vi "WaveGenerator.vi"(0 "Data array":dbl[][](array[numeric]), 1 "dt":dbl, 3 "TestLoops":i32, 5 "VMIC command":dbl[](array[numeric]), 9 "WaveDefineArray":T1[](array[typedef]) {"Enable" items=["不使能", "使能"]; "Wave" items=["0指令", "正弦波", "方波", "三角波", "常值", "波形数据", "白噪声", "正弦扫频", "梯度加载", "VMIC"]; "ChannelType" items=["标准波形跟踪"=1, "扫频测试"=2, "消除多余力"=3, "梯度加载"=4, "载荷谱跟踪"=5, "模拟输入跟踪"=9]; "ChannelStatus" items=["通道关", "位置通道", "加载通道"]}, 11 "Angle":dbl[](array[numeric]), 12 "AxisForce":dbl[](array[numeric]), 14 "LastVMICcommand":dbl[](array[numeric])) -> (4 "wave out 2":dbl[](array[numeric]), 6 "Command":dbl[](array[numeric]), 10 "Boolean":bool, 13 "VMICafterFilter":dbl[](array[numeric]), 15 "type out":dbl[](array[numeric]))   [LabVIEW 2014]
uses:
  ChannelCommand.ctl
  Control 1.ctl
  WaveType.ctl
  MoterEnable.ctl
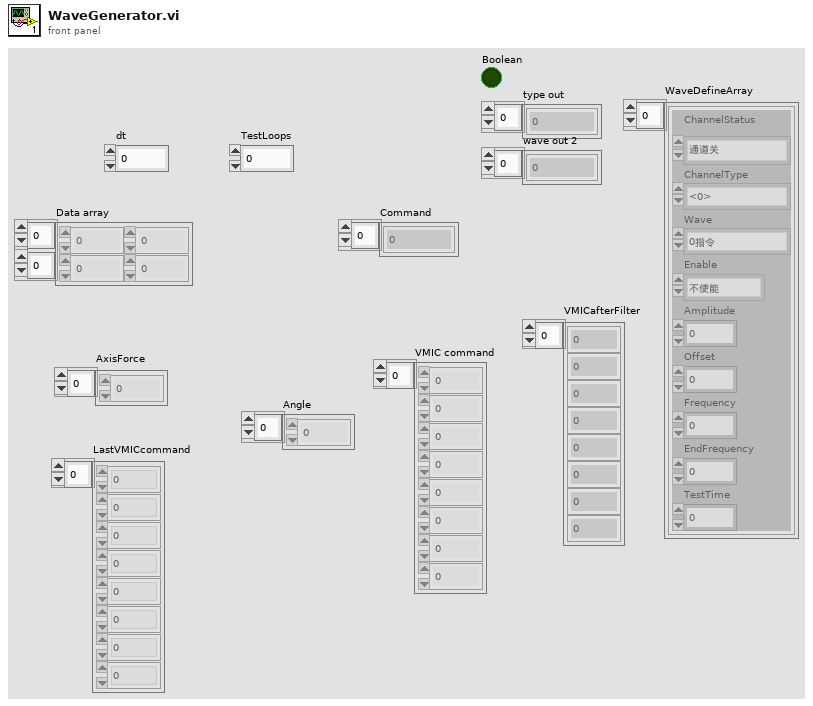
[diagram p1: front panel]
types:
  T1 = typedef "ChannelCommand.ctl" = cluster{"ChannelStatus":T2, "ChannelType":i32, "Wave":T3, "Enable":T4, "Amplitude":dbl, "Offset":dbl, "Frequency":dbl, "EndFrequency":dbl, "TestTime":dbl}
  T2 = typedef "Control 1.ctl" = i32
  T3 = typedef "WaveType.ctl" = i32
  T4 = typedef "MoterEnable.ctl" = u16
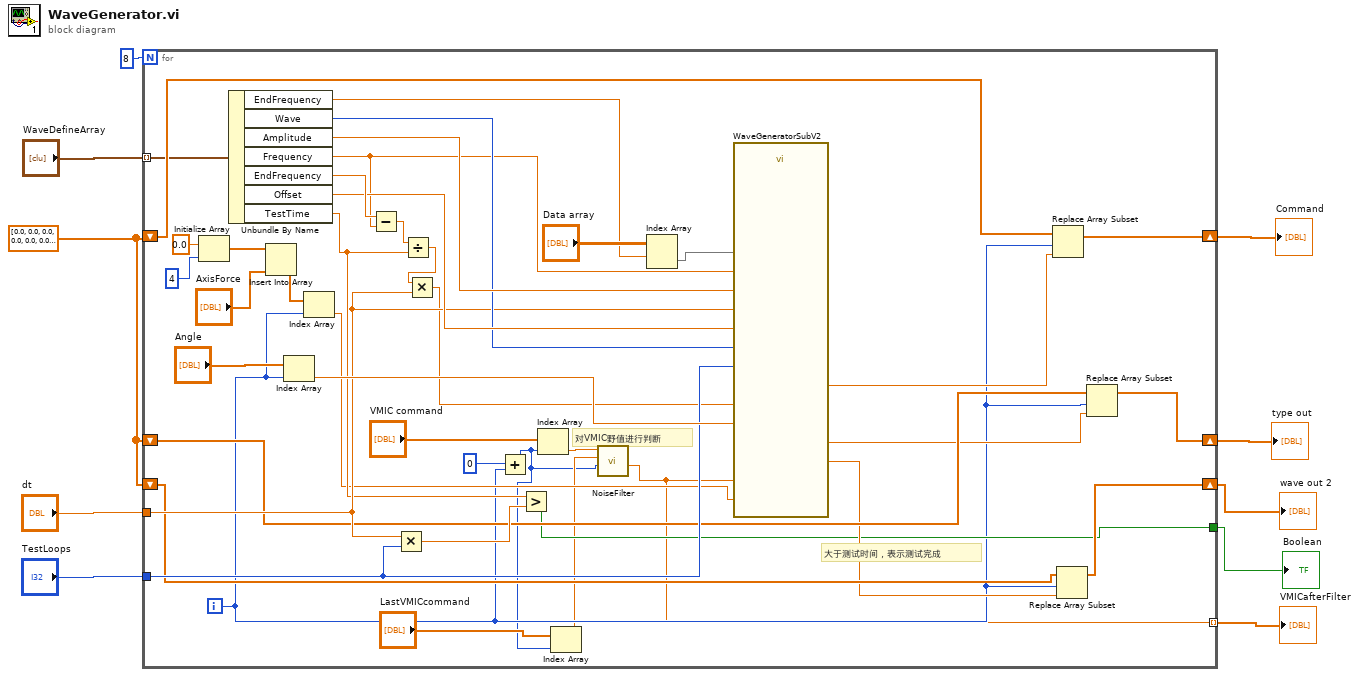
[diagram p0: block diagram]
diagram:
  w4 = dbl[] [0.0, 0.0, 0.0, 0.0, 0.0, 0.0, 0.0, 0.0]
  n1 = for {
    N: 8 -> [_]
    tunnel: "dt" -> [w36]
    tunnel: "TestLoops" -> [w37]
    tunnel: "WaveDefineArray" -> [w50] mode=indexing
    shift-right: [w51] -> w7
    shift-left: w4 -> [w52]
    tunnel: [w19] -> w3
    shift-right: [w32] -> w6
    shift-left: w4 -> [w31]
    shift-right: [w29] -> w5
    shift-left: w4 -> [w28]
    tunnel: [w11] -> w1 mode=indexing
    i -> [w17]
    # "对VMIC野值进行判断"
    # "大于测试时间，表示测试完成"
    n2 = Initialize Array(0.0 ("元素"), 4 ("维数大小")) -> (w21:dbl[])
    n3 = Unbundle By Name(w50) -> ("EndFrequency"=w48:dbl, "Wave"=w41:T3, "Amplitude"=w43:dbl, "Frequency"=w34:dbl, "EndFrequency"=w47:dbl, "Offset"=w42:dbl, "TestTime"=w33:dbl)
    n4 = Insert Into Array(array=w21, new element="AxisForce") -> (w20:dbl[])  [unwired: 1 in]
    n5 = Index Array(array="Angle", index=w17) -> (element=w39:dbl)
    n6 = Index Array(array=w20, index=w17) -> (element=w18:dbl)
    n7 = Subtract(x=w47, y=w34) -> (x-y=w46:dbl)
    n8 = Multiply(x=w36, y=w37) -> (x*y=w35:dbl)
    n9 = Divide(x=w46, y=w33) -> (x/y=w45:dbl)
    n10 = Multiply(x=w45, y=w36) -> (x*y=w25:dbl)
    n11 = Add(x=0, y=w17) -> (x+y=w12:i32)
    n12 = Greater?(x=w33, y=w35) -> (0:w19:bool)
    n13 = Index Array(array="VMIC command", index=w12) -> (element=w14:dbl)
    n14 = Index Array(array="LastVMICcommand", index=w12) -> (element=w13:dbl)
    n15 = call "NoiseFilter.vi"("loop"=w12, "lastCom"=w13, "TemCom"=w14) -> ("VmicOut"=w11:dbl)  [unwired: 8 in]
    n16 = Index Array(array="Data array", index (row)=w48) -> (element=w44:dbl[])  [unwired: 1 in]
    n17 = call "WaveGeneratorSubV2.vi"("Amplitude"=w43, "Wave"=w41, "ForceSample"=w18, "Data array"=w44, "Frequent"=w34, "Angle"=w39, "Offset"=w42, "deltaF"=w25, "VMIC"=w11, "dt"=w36, "TestLoops"=w37) -> ("Output"=w38:dbl, "Output 2"=w30:dbl, "waveout 3"=w27:dbl)  [unwired: 2 in]
    n18 = Replace Array Subset "Replace Array Subset"(array=w52, new element=w38, index=w17) -> (w51:dbl[])
    n19 = Replace Array Subset "Replace Array Subset"(array=w28, new element=w27, index=w17) -> (w29:dbl[])
    n20 = Replace Array Subset "Replace Array Subset"(array=w31, new element=w30, index=w17) -> (w32:dbl[])
  }
  "Command" <- w7
  "Boolean" <- w3
  "type out" <- w6
  "wave out 2" <- w5
  "VMICafterFilter" <- w1
